vi "Puma_Ground_Control_Station.vi"(0 "?":refnum<visa-resource-name>="COM1", 1 "?":u32=9600, 9 "XON":u8=17 format="%.0x", 14 "XOFF":u8=19 format="%.0x", 15 "?":u32=10000, 21 "?":bool=TRUE, 24 "?":u8=10 format="%.0x", 25 "bsize":u32=4096) -> ()   [LabVIEW 2014]
doc: "The Advanced Serial Read and Write example performs a Serial Port Read, a Serial Port Write, or a combination of these actions while setting some advanced serial features like buffer size, termination characters, and XON/XOFF flow control. The user selects the actions (read or write) on the front panel. If both are selected, the VI will write the data first, read the data and then close the VISA session that is opened to the port. \n\nThe parameters set for the serial port must match the parameters of the connected instrument or device. In this example, the bytes to read parameter specifies the number of bytes that the serial port reads. If there were more bytes at the port than the number specified in bytes to read, those bytes would not be read. Also, if you specify to read more bytes than the number of bytes actually read, you might receive a timeout error message.\n\nINSTRUCTIONS:\n1) Select the serial resource and configuration parameters (baud rate, data bits, parity, stop bits, flow control).\n2) Termination character can be enabled and set. Also, set the required input buffer size prior to running the example.\n3) Select the operations to be performed. \n4) Connect the serial port to your device. If no device is available, perform a loopback test by doing one of the following. Short pins 2 and 3 on a RS-232 cable or short pin 4 to pin 8 and pin 5 to pin 9 on a RS-485/422 cable. \n5) Run the VI to see the data read. (The \"read string\" will match the \"string to write\" if a loopback test was performed.)\n\nThis example exposes several advanced features that you may need for your application. Not all applications need all the features shown in this example. The input buffer size is likely an important setting that you want to control in your application. This example expands upon the flow control option for XON and XOFF, allowing the user to choose those control characters. The timeout parameter has been brought to the front panel so a user can specify the time period the VISA Read will wait for the number of bytes to read before timing out. Also, the user has several controls for the termination character, which is discussed later.\n\nNote that you can press the write and read buttons and change the bytes to read parameters on the fly, while the example is running. However, you must stop the example to change the other configuration parameters after the example has started running, and then run again.\n\nSet the I/O buffer size slightly higher the amount of data you expect to receive. This is very important for applications that don't use flow control, as you may lose characters if the receive buffer overflows.\n\nSetting the timeout period ensures that the operation returns with a timeout error if the operation cannot be performed in the specified time period. \n\nSome devices require a termination character in order to identify the end of command strings. Some devices send a termination character to signify the end of data to be read. \n\nThis example shows how you can end the Read operation once a termination character is detected in the buffer and/or append a termination character at the end of the Write data. To enable the Read to end on a termination character, use the VISA Configure Serial Port or use the VISA Properties Serial End Mode for Reads, Termination Character Enable, and Termination Character. To end the Write with a termination character, use the VISA Properties Serial End Mode for Writes, the Send End Enable, and Termination Character. In this example, the same termination character is used for both the Read and the Write. You can specify two different characters for your application, if desired.\n\nYour application may require specific characters for the XON/XOFF Flow Control. You can specify these characters with the VISA Properties Flow Control XOFF Character and Flow Control XON Character. Note that if the standard XON and XOFF characters are used, then decimal 17 and 19 are unavailable for data values. Remember that using flow control and setting an adequate buffer size allow you to prevent buffer overflows."
uses:
  <vilib>/Instr/_visa.llb/VISA Configure Serial Port (Instr).vi
panel:
  out "soft kill ind":bool
  out "dump fuel ind":bool
  out "abort ind":bool
  out "run ind":bool
  out "av6-t ind":bool
  out "Control input":bool
  out "return yes on a completed input":bool
  out "Control (on/off)":bool
  out "PT 7":dbl
  out "PT7":dbl
  out "PT6":dbl
  out "PT5":dbl
  out "PT4":dbl
  out "PT3":dbl
  out "PT2":dbl
  out "PT1":dbl
  out "TC6":dbl
  out "TC5":dbl
  out "TC4":dbl
  out "TC3":dbl
  out "TC2":dbl
  out "TC1":dbl
  out "Output":string
  in  "?":enum32{"Check Out's", "Test"}(tab)
  in  "Tank ISO / AV5-T":bool
  in  "DValve / AV6-T":bool
  in  "Ullage ISO / FC-U":bool
  in  "UDump / FO-U":bool
  in  "Flight Control Board":bool
  in  "Safety":bool
  in  "Test Run":bool
  in  "Reset Control":bool
  in  "Primary Safety":bool
  out "?":bool
  out "?":bool
  out "?":bool
  out "?":bool
  in  "Primary Safety TEST Primary Safety":bool
  in  "Soft Kill":bool
  in  "Extra Switch":bool
  in  "Reset FC":bool
  in  "PixHawk":bool
  in  "Flight Control":bool
  in  "Safety":bool
  in  "Takeoff":bool
  in  "abort":bool
  out "?":dbl(graph)
  in  "Send Command":bool=TRUE
  in  "Manual":string="*IDN?"
  in  "?":bool=TRUE
  in  "bytes to read 2":u32=1000
  out "?":u32
  out "?":string[](array[string])
  out "?":string[](array[string])
  out "?":T1(graph)
  out "Voltage Sensor":dbl
  out "PT 1":dbl
  out "PT 2":dbl
  out "PT 3":dbl
  out "PT 4":dbl
  out "PT 5":dbl
  out "PT 6":dbl
  out "TC 1":dbl
  out "TC 2":dbl
  out "TC 3":dbl
  out "TC 4":dbl
  out "TC 5":dbl
  out "TC 6":dbl
  in  "dump fuel":bool
  in  "?":enum32{"PT", "TC", "Test"}(tab)
  in  "?":T2(tab)
  out "PT 1":dbl(graph)
  out "PT 2":dbl(graph)
  out "PT 3":dbl(graph)
  out "PT 4":dbl(graph)
  out "PT 5":dbl(graph)
  out "PT 6":dbl(graph)
  out "PT 7":dbl(graph)
  in  "?":T3(tab)
  out "TC 1":dbl(graph)
  out "TC 2":dbl(graph)
  out "TC 3":dbl(graph)
  out "TC 4":dbl(graph)
  out "TC 5":dbl(graph)
  out "TC 6":dbl(graph)
  out "?":bool
  out "String":string
  in  "String 3":string
  in  "Turn Off":bool
  in  "?":bool=TRUE
  in  "?":bool
  in  "Av-6Tt":bool
  in  "?":bool
  in  "?":bool
  out "AV4-T":bool
  out "AV3-T":bool
  out "AV2-T":bool
  out "AV1-T":bool
  out "AV6-T":bool
  out "AV5-T":bool
  out "FO-U":bool
  out "FC-U":bool
  out "?":dbl(slide) scale=0.2..200.0
  # "FC-U"
  # "FO-U"
  # "AV1-T"
  # "AV2-T"
  # "AV3-T"
  # "AV4-T"
  # "AV5-T"
  # "AV6-T"
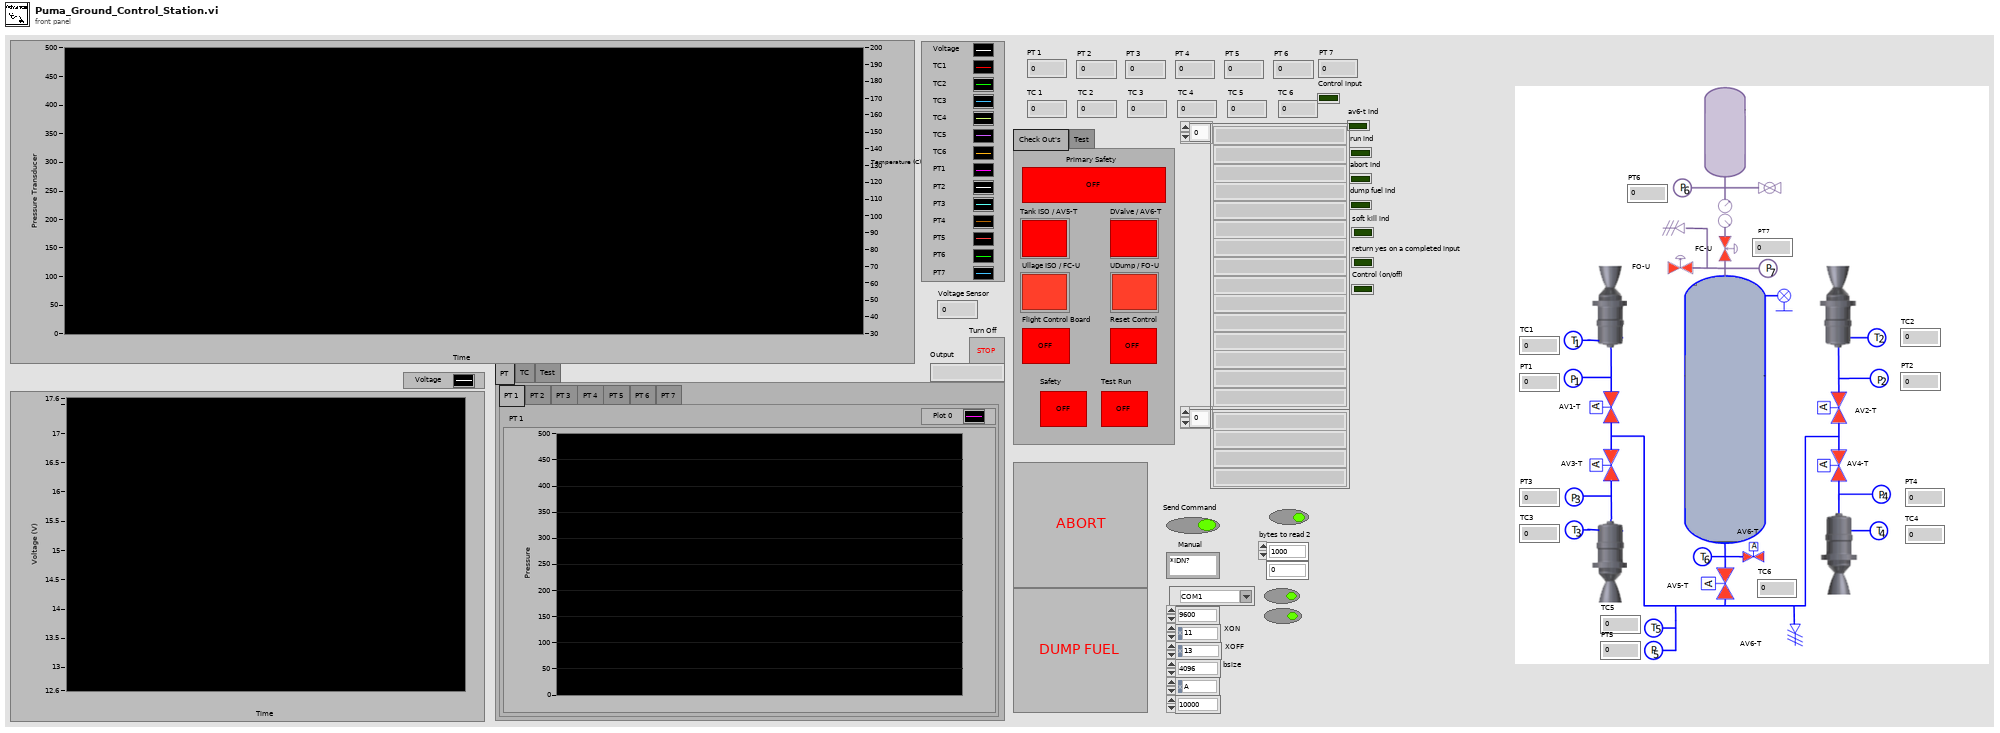
[diagram p1: front panel]
types:
  T1 = cluster{dbl, dbl, dbl, dbl, dbl, dbl, dbl, dbl, dbl, dbl, dbl, dbl, dbl, dbl}
  T2 = enum32{"PT 1", "PT 2", "PT 3", "PT 4", "PT 5", "PT 6", "PT 7"}
  T3 = enum32{"TC 1", "TC 2", "TC 3", "TC 4", "TC 5", "TC 6"}
  T4 = cluster{"Read Access":enum8{"Allowed", "Required", "None"}, "Write Access":enum8{"Allowed", "Required", "None"}}
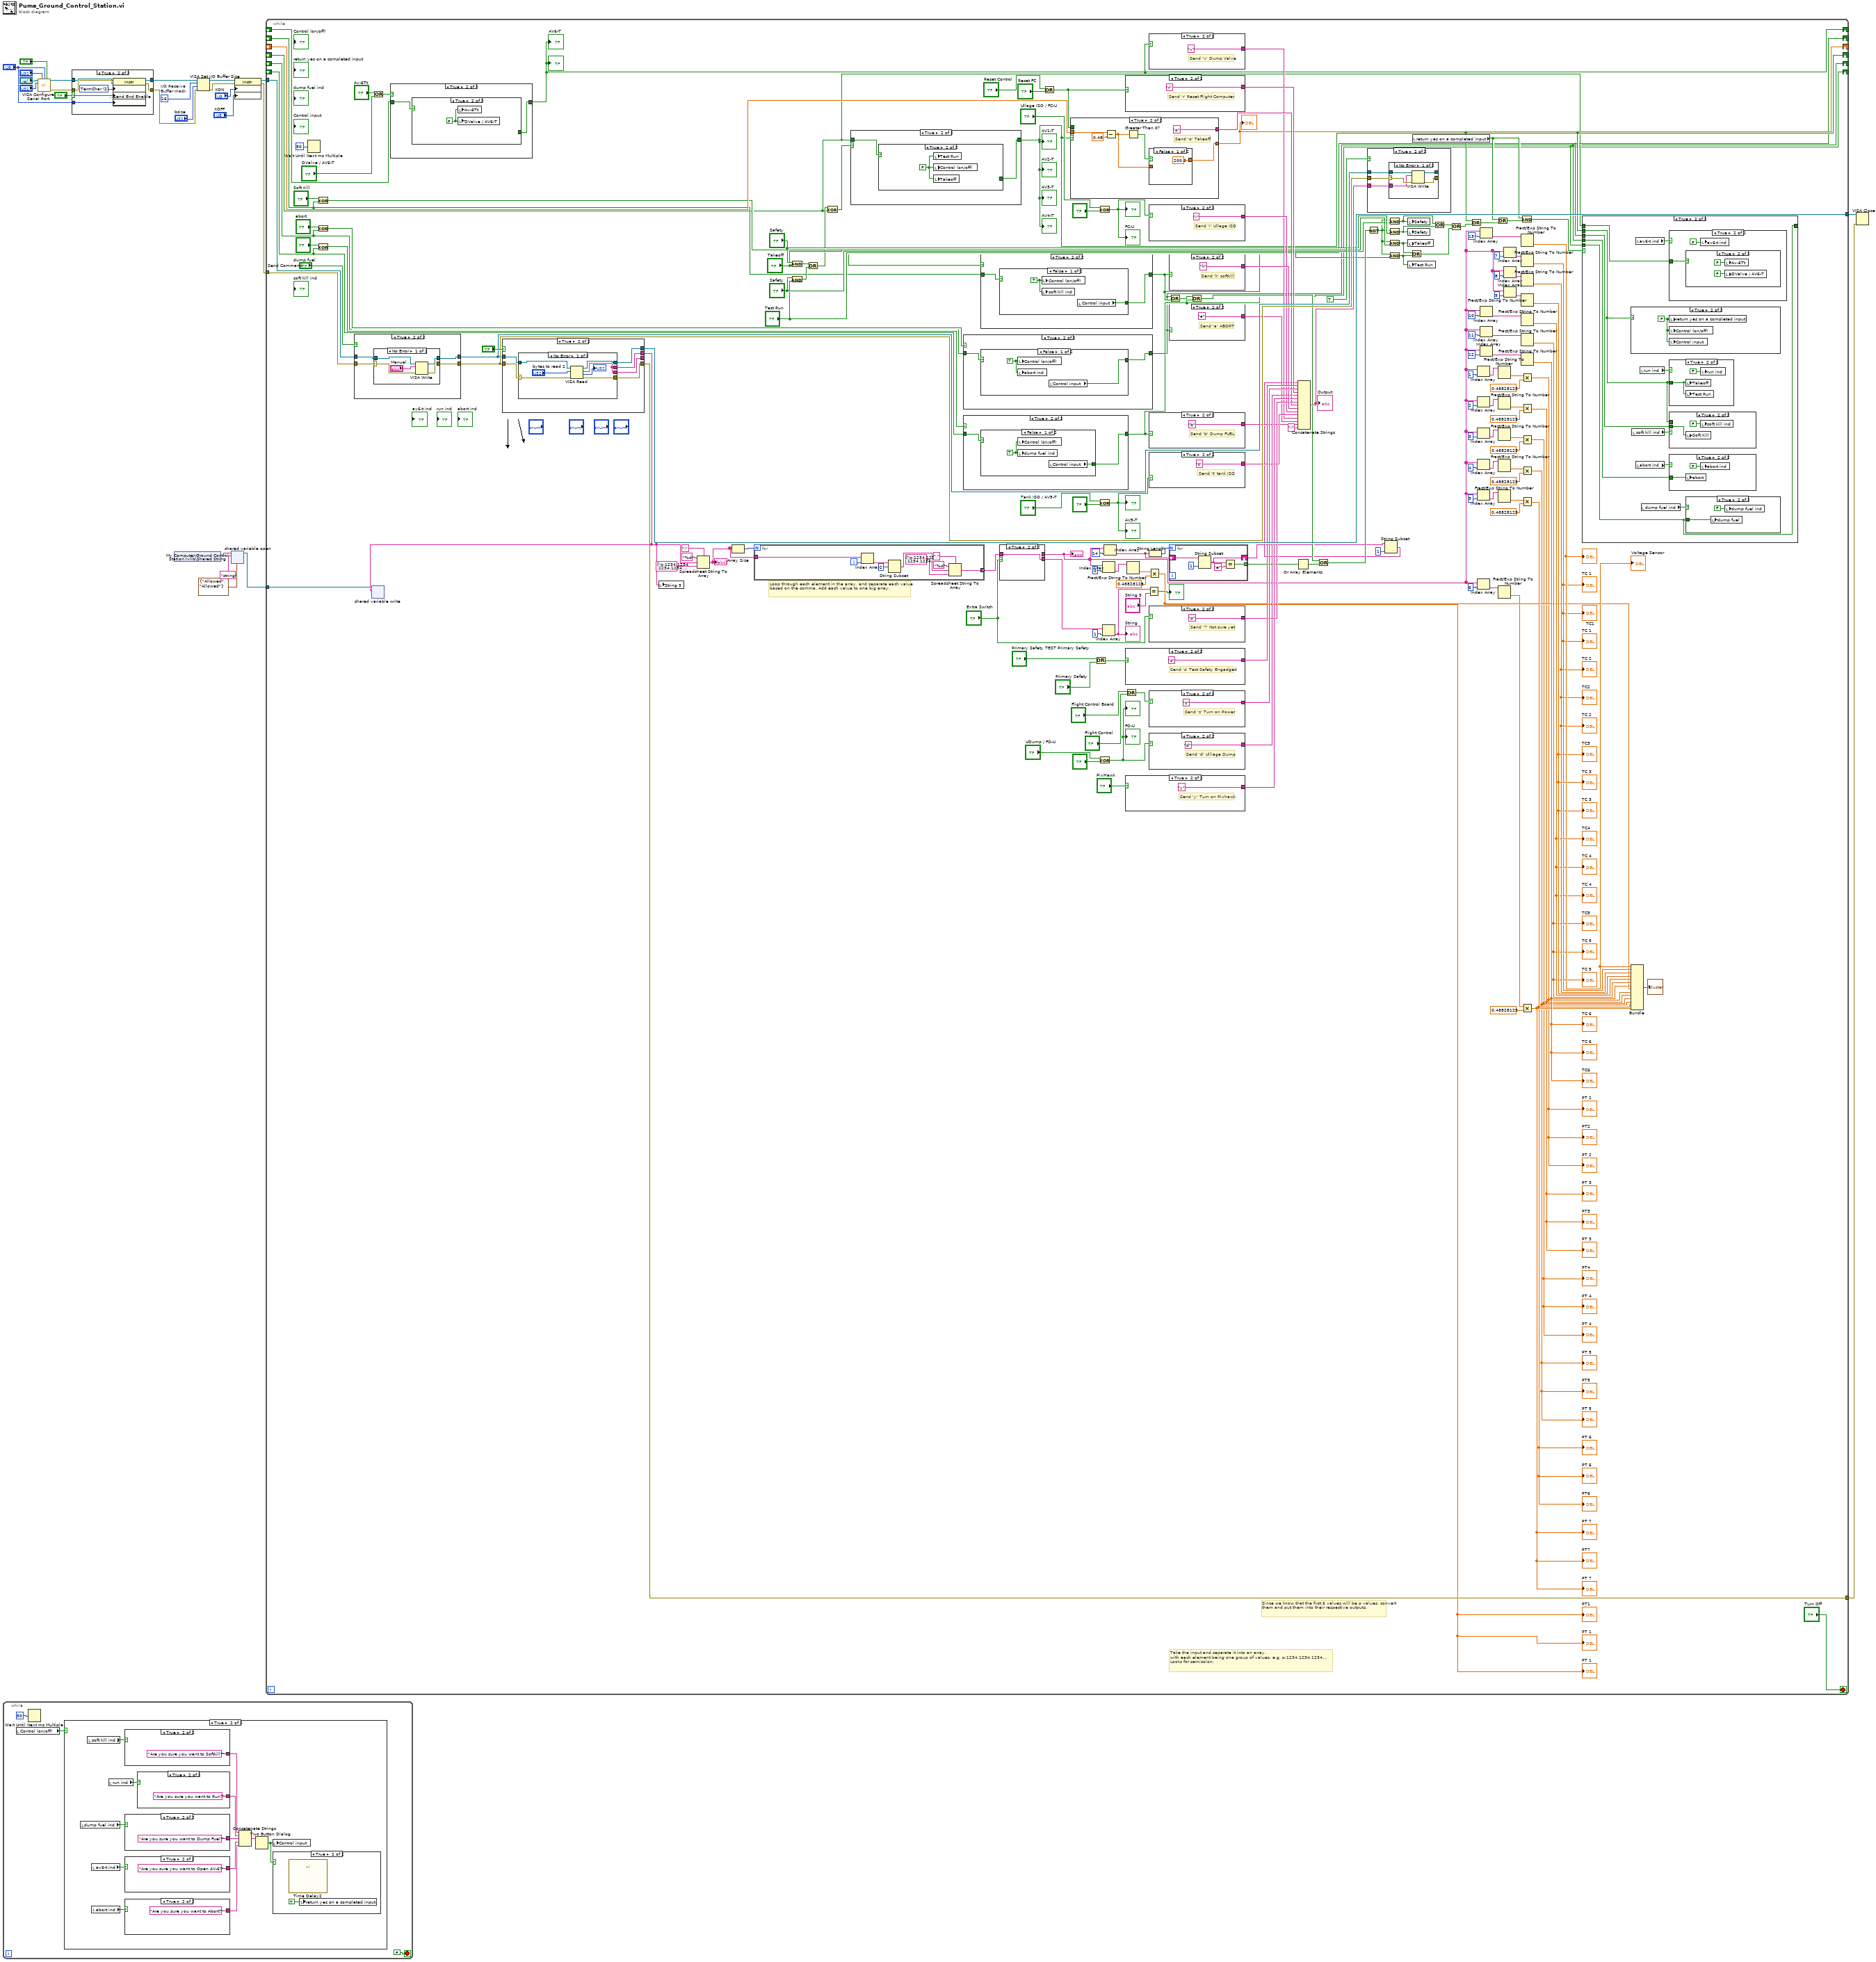
[diagram p0: block diagram]
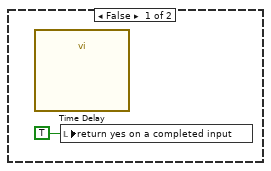
[diagram p8: hidden frame]
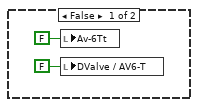
[diagram p11: hidden frame]
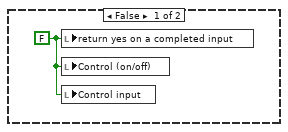
[diagram p16: hidden frame]
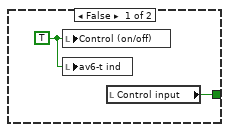
[diagram p18: hidden frame]
diagram:
  w20 = u16 16  # I/O Receive Buffer mask
  n1 = while {
    stop <- FALSE stop-if-true
    n2 = local read "Control (on/off)"() -> (w27:bool)
    n3 = Wait Until Next ms Multiple(millisecond multiple=u32 50 ("milliseconds to wait")) -> ()  [unwired: 1 out]
    n4 = case shown="True" w27 {
      frame False {
      }
      frame True {
        n5 = local read "dump fuel ind"() -> (w36:bool)
        n6 = local read "soft kill ind"() -> (w34:bool)
        n7 = local read "av6-t ind"() -> (w37:bool)
        n8 = local read "abort ind"() -> (w38:bool)
        n9 = local read "run ind"() -> (w35:bool)
        n10 = case shown="True" w34 {
          tunnel: [_ "Are you sure you want to Softkill?"] -> w29
          frame False {
          }
          frame True {
          }
        }
        n11 = case shown="True" w36 {
          tunnel: [_ "Are you sure you want to Dump Fuel?"] -> w31
          frame False {
          }
          frame True {
          }
        }
        n12 = case shown="True" w37 {
          tunnel: [_ "Are you sure you want to Open AV-6?"] -> w32
          frame False {
          }
          frame True {
          }
        }
        n13 = case shown="True" w38 {
          tunnel: [_ "Are you sure you want to Abort?"] -> w33
          frame False {
          }
          frame True {
          }
        }
        n14 = case shown="True" w35 {
          tunnel: [_ "Are you sure you want to Run?"] -> w30
          frame False {
          }
          frame True {
          }
        }
        n15 = Concatenate Strings(w29, w30, w31, w32, w33) -> (w28:string)
        n16 = Two Button Dialog(message=w28) -> (T button?=w39:bool)  [unwired: 2 in]
        n17 = local write "Control input"(w39) -> ()
        n18 = case shown="True" w39 {
          frame False {
            n19 = call "Time Delay"() -> ()  [unwired: 11 in, 1 out]
            n20 = local write "return yes on a completed input"(TRUE) -> ()
          }
          frame True {
            n21 = call "Time Delay2"() -> ()  [unwired: 11 in, 1 out]
            n22 = local write "return yes on a completed input"(TRUE) -> ()
          }
        }
      }
    }
  }
  n23 = call-poly "VISA Configure Serial Port"("VISA resource name"="?", "timeout (10sec)"="?", "termination char\n(0xA = '\\n' = LF)"="?", "Enable Termination\nChar (T)"="?", "baud rate (9600)"="?") -> ("VISA resource name out"=w9:refnum<visa-resource-name>, "error out"=w12:errorcluster)  [unwired: 5 in, 4 out]
  n24 = case shown="True" "?" {
    selector: "?" -> [_ w49]
    tunnel: w9 -> [w47 w55]
    tunnel: w12 -> [w48 w54]
    tunnel: [w47 w53] -> w10
    tunnel: [w48 w52] -> w11
    tunnel: "?" -> [_ w50]
    frame False {
    }
    frame True {
      w51 = u16 2 items=["None", "LastBit", "TermChar", "Break"] ("Serial Settings:Serial End Mode for Writes")
      n25 = property class="Instr"(reference=w55, error in=w54, "Serial Settings:End Mode for Writes"=w51, "Message Based Settings:Send End Enable"=w49, "Message Based Settings:Termination Character"=w50) -> (reference out=w53:refnum<visa-resource-name>, error out=w52:errorcluster)
    }
  }
  n26 = shared-variable "My Computer\\Ground Control Station.lvlib\\Shared String"() -> (w2:string)  [unwired: 1 in, 1 out]
  n27 = VISA Set I/O Buffer Size(VISA resource name=w10, mask (16)=w20, size (4096)="bsize", error in (no error)=w11) -> (VISA resource name out=w16:refnum<visa-resource-name>, error out=w15:errorcluster)
  n28 = shared-variable-open(w2, "string", T4 {"Read Access"=enum."Allowed", "Write Access"=enum."Allowed"} ("access")) -> (w1:refnum<k21>)  [unwired: 1 in, 1 out]
  n29 = property class="Instr"(reference=w16, error in=w15, "Serial Settings:Flow Control XON Character"="XON", "Serial Settings:Flow Control XOFF Character"="XOFF") -> (reference out=w8:refnum<visa-resource-name>, error out=w7:errorcluster)
  n30 = while {
    tunnel: w8 -> [w191]
    tunnel: w7 -> [w190]
    tunnel: [w189] -> w6
    tunnel: [w58] -> w5
    shift-right: [w149] -> _
    shift-left: _ -> [w148]
    shift-right: [w84] -> _
    shift-left: _ -> [w66]
    shift-right: [w74] -> _
    shift-left: _ -> [w75]
    shift-right: [w64] -> _
    shift-left: _ -> [w91]
    shift-right: [w65] -> _
    shift-left: _ -> [w88]
    shift-right: [w67] -> _
    shift-left: _ -> [w70]
    tunnel: w1 -> [w57]
    stop <- "Turn Off" stop-if-true
    # "Since we know that the first 6 values will be p values, convert them and put them into their respective outputs."
    # "Loop through each element in the array, and separate each value\nbased on the comma. Add each value to one big array."
    # "Take the input and separate it into an array,\nwith each element being one group of values, e.g. p:1234,1234,1234...\nLooks for semicolon."
    n31 = Wait Until Next ms Multiple(millisecond multiple=u32 50 ("milliseconds to wait")) -> ()  [unwired: 1 out]
    n32 = Exclusive Or(1:w70, 2:"Soft Kill") -> (0:w68:bool)
    n33 = Exclusive Or(1:w91, 2:"abort") -> (0:w93:bool)
    n34 = Exclusive Or(1:w88, 2:"dump fuel") -> (0:w90:bool)
    n35 = case shown="True" "Send Command" {
      tunnel: [w322 w326] -> w184
      tunnel: [w321 w325] -> w183
      tunnel: w191 -> [w322 w324]
      tunnel: w190 -> [w321 w323]
      frame False {
      }
      frame True {
        n36 = case shown="No Error" w323 {
          selector: w323 -> [w327 w333]
          tunnel: [w331 w332] -> w326
          tunnel: [w330 w333] -> w325
          tunnel: w324 -> [w328 w332]
          frame No Error {
            n37 = VISA Write(VISA resource name=w328, write buffer="Manual", error in (no error)=w327) -> (VISA resource name out=w331:refnum<visa-resource-name>, error out=w330:errorcluster)  [unwired: 1 out]
          }
          frame Error {
          }
        }
      }
    }
    n38 = Or(x="Av-6Tt", y="DValve / AV6-T") -> (x .or. y?=w71:bool)
    n39 = case shown="True" w71 {
      tunnel: [w251 w252] -> w74
      tunnel: w75 -> [w251 w253]
      frame False {
      }
      frame True {
        n40 = case shown="True" w253 {
          tunnel: [w255 _] -> w252
          frame False {
            w254 = TRUE
            n41 = local write "Control (on/off)"(w254) -> ()
            n42 = local write "av6-t ind"(w254) -> ()
            n43 = local read "Control input"() -> (w255:bool)
          }
          frame True {
            w256 = FALSE
            n44 = local write "Av-6Tt"(w256) -> ()
            n45 = local write "DValve / AV6-T"(w256) -> ()
          }
        }
      }
    }
    "AV6-T" <- w74
    "?" <- w74
    n46 = case shown="True" "?" {
      tunnel: w183 -> [w334 w339]
      tunnel: w184 -> [w335 w338]
      tunnel: [w334 w341] -> w58
      tunnel: [w335 w340] -> w189
      tunnel: [_ w337] -> _
      tunnel: [_ w336] -> w56
      frame False {
      }
      frame True {
        n47 = case "Read bytes from port." shown="No Error" w339 {
          selector: w339 -> [w344 w349]
          tunnel: [w347 w349] -> w341
          tunnel: [w348 w350] -> w340
          tunnel: w338 -> [w345 w350]
          tunnel: [w342 _] -> w337
          tunnel: [w342 _] -> w336
          frame No Error {
            n48 = VISA Read(VISA resource name=w345, byte count="bytes to read 2", error in (no error)=w344) -> (VISA resource name out=w348:refnum<visa-resource-name>, read buffer=w342:string, return count=→"?":u32, error out=w347:errorcluster)
          }
          frame Error {
            # "Error occurred \nreading Bytes at \nSerial Port"
          }
        }
      }
    }
    n49 = shared-variable-write(w57, w56) -> ()  [unwired: 1 in, 2 out]
    n50 = local write "String 3"(w56) -> ()
    n51 = Spreadsheet String To Array(delimiter (Tab)=";", format string="%d", spreadsheet string=w56, array type (2D Dbl)=string[] ["p:1234.1234.1234.1234,1234,1234", "t:1234,1234,1234"] ("Array of Strings 3")) -> (array=w217:string[])
    "?" <- w217
    n52 = Array Size(array=w217) -> (size(s)=w218:i32)
    n53 = for {
      N: w218 -> [_]
      tunnel: w217 -> [w359]
      tunnel: [w351] -> w112 mode=concatenating
      i -> [w358]
      n54 = Index Array(array=w359, index=w358) -> (element=w354:string)
      n55 = String Subset(string=w354, offset (0)=2) -> (substring=w352:string)  [unwired: 1 in]
      n56 = Spreadsheet String To Array(delimiter (Tab)=",", format string="%d", spreadsheet string=w352, array type (2D Dbl)=string[] ["p:1234.1234.1234.1234,1234,1234", "t:1234,1234,1234"] ("Array of Strings 3")) -> (array=w351:string[])
    }
    n57 = And(x="Safety", y="Takeoff") -> (x .and. y?=w169:bool)
    n58 = And(x="Safety", y="Test Run") -> (x .and. y?=w170:bool)
    n59 = Or(x=w169, y=w170) -> (x .or. y?=w96:bool)
    n60 = Exclusive Or(1:w66, 2:w96) -> (0:w95:bool)
    n61 = case shown="True" w95 {
      tunnel: [w273 w275] -> w84
      tunnel: w66 -> [w273 w274]
      frame False {
      }
      frame True {
        n62 = case shown="True" w274 {
          tunnel: [w277 _] -> w275
          frame False {
            w276 = TRUE
            n63 = local write "Control (on/off)"(w276) -> ()
            n64 = local write "run ind"(w276) -> ()
            n65 = local read "Control input"() -> (w277:bool)
          }
          frame True {
            w278 = FALSE
            n66 = local write "Test Run"(w278) -> ()
            n67 = local write "Control (on/off)"(w278) -> ()
            n68 = local write "Takeoff"(w278) -> ()
          }
        }
      }
    }
    "AV1-T" <- w84
    "AV4-T" <- w84
    "AV2-T" <- w84
    "AV3-T" <- w84
    n69 = case shown="True" w93 {
      tunnel: [w267 w269] -> w64
      tunnel: w91 -> [w267 w268]
      frame False {
      }
      frame True {
        n70 = case shown="False" w268 {
          tunnel: [w270 FALSE ("T button?")] -> w269
          frame False {
            w271 = TRUE
            n71 = local write "Control (on/off)"(w271) -> ()
            n72 = local write "abort ind"(w271) -> ()
            n73 = local read "Control input"() -> (w270:bool)
          }
          frame True {
          }
        }
      }
    }
    n74 = case shown="True" w90 {
      tunnel: [w262 w264] -> w65
      tunnel: w88 -> [w262 w263]
      frame False {
      }
      frame True {
        n75 = case shown="False" w263 {
          tunnel: [w266 _] -> w264
          frame False {
            w265 = TRUE
            n76 = local write "Control (on/off)"(w265) -> ()
            n77 = local write "dump fuel ind"(w265) -> ()
            n78 = local read "Control input"() -> (w266:bool)
          }
          frame True {
          }
        }
      }
    }
    n79 = case shown="True" w68 {
      tunnel: [w257 w259] -> w67
      tunnel: w70 -> [w257 w258]
      frame False {
      }
      frame True {
        n80 = case shown="False" w258 {
          tunnel: [w260 _] -> w259
          frame False {
            w261 = TRUE
            n81 = local write "Control (on/off)"(w261) -> ()
            n82 = local write "soft kill ind"(w261) -> ()
            n83 = local read "Control input"() -> (w260:bool)
          }
          frame True {
          }
        }
      }
    }
    n84 = case shown="True" "Extra Switch" {
      tunnel: w112 -> [w284 w285]
      tunnel: [w284 _] -> w114
      tunnel: [_ w285] -> w111
      frame False {
      }
      frame True {
      }
    }
    "?" <- w114
    n85 = Or(x="Reset Control", y="Reset FC") -> (x .or. y?=w150:bool)
    n86 = case shown="True" w84 {
      tunnel: [_ "o" ("write buffer")] -> w175
      tunnel: w148 -> [w295 w303]
      tunnel: [w296 w299] -> w149
      tunnel: w150 -> [w294 _]
      frame False {
        n87 = case shown="False" w294 {
          tunnel: [w297 200.0] -> w296
          tunnel: w295 -> [w297 _]
          frame False {
          }
          frame True {
          }
        }
      }
      frame True {
        # "Send 'o' Takeoff"
        n88 = Subtract(x=w303, y=0.48) -> (x-y=w300:dbl)
        n89 = Greater Than 0?(x=w300) -> (x > 0?=w301:bool)
        n90 = case shown="False" w301 {
          tunnel: w300 -> [_ w306]
          tunnel: [200.0 w306] -> w299
          frame False {
          }
          frame True {
          }
        }
      }
    }
    "?" <- w149
    n91 = Or(x="Primary Safety TEST Primary Safety", y="Primary Safety") -> (x .or. y?=w136:bool)
    n92 = Exclusive Or(1:"?", 2:"Ullage ISO / FC-U") -> (0:w139:bool)
    "FC-U" <- w139
    "?" <- w139
    n93 = Exclusive Or(1:"?", 2:"Tank ISO / AV5-T") -> (0:w142:bool)
    "AV5-T" <- w142
    "?" <- w142
    n94 = Exclusive Or(1:"?", 2:"UDump / FO-U") -> (0:w145:bool)
    "FO-U" <- w145
    "?" <- w145
    n95 = Index Array(array=w114, index=0) -> (element=w210:string)
    n96 = Index Array(array=w111, index=1) -> (element=w110:string)
    "String" <- w110
    n97 = Index Array(array=w114, index=14) -> (element=w59:string)
    n98 = case shown="True" w150 {
      tunnel: [_ "r" ("write buffer")] -> w179
      frame False {
      }
      frame True {
        # "Send 'r' Reset Flight Computer"
      }
    }
    n99 = case shown="True" w136 {
      tunnel: [_ "s" ("write buffer")] -> w182
      frame False {
      }
      frame True {
        # "Send 's' Test Safety Engadged"
      }
    }
    n100 = case shown="True" "PixHawk" {
      tunnel: [_ "y" ("write buffer")] -> w177
      frame False {
      }
      frame True {
        # "Send 'y' Turn on Pixhawk"
      }
    }
    n101 = Or(x="Flight Control Board", y="Flight Control") -> (x .or. y?=w166:bool)
    n102 = Fract/Exp String To Number(string=w210) -> (number=w131:dbl)  [unwired: 3 in, 1 out]
    n103 = Equal?(x=w110, y="String 3") -> (x = y?=→"?":bool)
    n104 = Multiply(x=w131, y=0.48828125) -> (x*y=w130:dbl)
    "PT 1" <- w130
    "PT 1" <- w130
    "PT1" <- w130
    n105 = case shown="True" w74 {
      tunnel: [_ "v" ("write buffer")] -> w162
      frame False {
      }
      frame True {
        # "Send 'v' Dump Valve"
      }
    }
    n106 = case shown="True" w139 {
      tunnel: [_ "i" ("write buffer")] -> w164
      frame False {
      }
      frame True {
        # "Send 'i' Ullage ISO"
      }
    }
    n107 = case shown="True" w65 {
      tunnel: [_ "b" ("write buffer")] -> w161
      frame False {
      }
      frame True {
        # "Send 'b' Dump FUEL"
      }
    }
    n108 = case shown="True" w142 {
      tunnel: [_ "t" ("write buffer")] -> w163
      frame False {
      }
      frame True {
        # "Send 't' tank ISO"
      }
    }
    n109 = String Length(string=w59) -> (length=w106:i32)
    n110 = case shown="True" "Extra Switch" {
      tunnel: [_ "p" ("write buffer")] -> w176
      frame False {
      }
      frame True {
        # "Send '?' Not sure yet"
      }
    }
    n111 = case shown="True" w166 {
      tunnel: [_ "z" ("write buffer")] -> w180
      frame False {
      }
      frame True {
        # "Send 'z' Turn on Power"
      }
    }
    n112 = case shown="True" w145 {
      tunnel: [_ "d" ("write buffer")] -> w165
      frame False {
      }
      frame True {
        # "Send 'd' Ulliage Dump"
      }
    }
    n113 = case shown="True" w67 {
      tunnel: [_ "k" ("write buffer")] -> w178
      frame False {
      }
      frame True {
        # "Send 'k' softkill"
      }
    }
    n114 = Or(x=w64, y=w67) -> (x .or. y?=w94:bool)
    n115 = case shown="True" w64 {
      tunnel: [_ "a" ("write buffer")] -> w160
      frame False {
      }
      frame True {
        # "Send 'a' ABORT"
      }
    }
    n116 = for {
      N: w106 -> [_]
      shift-right: [w281] -> w61
      shift-left: w59 -> [w280]
      tunnel: [w279] -> w105 mode=indexing
      n117 = String Subset(string=w280, length (rest)=1 ("length (rest)")) -> (substring=w281:string)  [unwired: 1 in]
      n118 = Equal?(x=w281, y="e") -> (x = y?=w279:bool)
    }
    n119 = Or(x=w94, y=w65) -> (x .or. y?=w103:bool)
    n120 = Or Array Elements(Boolean array=w105) -> (logical OR=w104:bool)
    n121 = Or(x=w103, y=w104) -> (x .or. y?=w102:bool)
    n122 = Not(x=w102) -> (.not. x?=w98:bool)
    n123 = String Subset(string=w61, length (rest)=1 ("length (rest)")) -> (substring=w63:string)  [unwired: 1 in]
    n124 = Concatenate Strings(w63, w182, w180, w179, w165, w177, w176, w175, w178, w164, w163, w162, w160, w161, ";" ("string")) -> (w173:string)
    "Output" <- w173
    n125 = case shown="True" TRUE {
      tunnel: w184 -> [_ w313]
      tunnel: w183 -> [_ w312]
      tunnel: w173 -> [_ w311]
      frame False {
      }
      frame True {
        n126 = case shown="No Error" w312 {
          selector: w312 -> [w315 w320]
          tunnel: [w318 w319] -> _
          tunnel: [w317 w320] -> _
          tunnel: w313 -> [w316 w319]
          tunnel: w311 -> [w314 _]
          frame No Error {
            n127 = VISA Write(VISA resource name=w316, write buffer=w314, error in (no error)=w315) -> (VISA resource name out=w318:refnum<visa-resource-name>, error out=w317:errorcluster)  [unwired: 1 out]
          }
          frame Error {
          }
        }
      }
    }
    n128 = And(x=w98, y="Safety") -> (x .and. y?=w79:bool)
    n129 = And(x=w98, y="Safety") -> (x .and. y?=w78:bool)
    n130 = And(x=w98, y="Takeoff") -> (x .and. y?=w77:bool)
    n131 = And(x=w98, y="Test Run") -> (x .and. y?=w76:bool)
    n132 = local write "Safety"(w79) -> ()
    n133 = local write "Safety"(w78) -> ()
    n134 = local write "Takeoff"(w77) -> ()
    n135 = local write "Test Run"(w76) -> ()
    n136 = Or(x=w77, y=w76) -> (x .or. y?=w81:bool)
    n137 = local read "return yes on a completed input"() -> (w86:bool)
    n138 = Or(x=w79, y=w78) -> (x .or. y?=w82:bool)
    n139 = Or(x=w82, y=w81) -> (x .or. y?=w80:bool)
    n140 = Or(x=w84, y=w80) -> (x .or. y?=w83:bool)
    n141 = Index Array(array=w114, index=1) -> (element=w209:string)
    n142 = Index Array(array=w114, index=2) -> (element=w208:string)
    n143 = Index Array(array=w114, index=3) -> (element=w207:string)
    n144 = Index Array(array=w114, index=4) -> (element=w206:string)
    n145 = Index Array(array=w114, index=5) -> (element=w205:string)
    n146 = Index Array(array=w114, index=6) -> (element=w152:string)
    n147 = Index Array(array=w114, index=13) -> (element=w187:string)
    n148 = Index Array(array=w114, index=10) -> (element=w195:string)
    n149 = Index Array(array=w114, index=11) -> (element=w194:string)
    n150 = Index Array(array=w114, index=12) -> (element=w193:string)
    n151 = Or(x=w86, y=w83) -> (x .or. y?=w87:bool)
    n152 = Fract/Exp String To Number(string=w209) -> (number=w116:dbl)  [unwired: 3 in, 1 out]
    n153 = Fract/Exp String To Number(string=w208) -> (number=w119:dbl)  [unwired: 3 in, 1 out]
    n154 = Fract/Exp String To Number(string=w207) -> (number=w122:dbl)  [unwired: 3 in, 1 out]
    n155 = Fract/Exp String To Number(string=w206) -> (number=w125:dbl)  [unwired: 3 in, 1 out]
    n156 = Fract/Exp String To Number(string=w205) -> (number=w134:dbl)  [unwired: 3 in, 1 out]
    n157 = Fract/Exp String To Number(string=w152) -> (number=w128:dbl)  [unwired: 3 in, 1 out]
    n158 = Index Array(array=w114, index=7) -> (element=w199:string)
    n159 = Index Array(array=w114, index=8) -> (element=w198:string)
    n160 = Index Array(array=w114, index=9) -> (element=w197:string)
    n161 = And(x=w86, y=w87) -> (x .and. y?=w85:bool)
    n162 = Fract/Exp String To Number(string=w187) -> (number=w186:dbl)  [unwired: 3 in, 1 out]
    "Voltage Sensor" <- w186
    "?" <- w186
    n163 = Fract/Exp String To Number(string=w199) -> (number=w153:dbl)  [unwired: 3 in, 1 out]
    "TC 1" <- w153
    "TC 1" <- w153
    "TC1" <- w153
    n164 = Fract/Exp String To Number(string=w198) -> (number=w158:dbl)  [unwired: 3 in, 1 out]
    "TC 2" <- w158
    "TC 2" <- w158
    "TC2" <- w158
    n165 = Fract/Exp String To Number(string=w197) -> (number=w157:dbl)  [unwired: 3 in, 1 out]
    "TC 3" <- w157
    "TC 3" <- w157
    "TC3" <- w157
    n166 = Fract/Exp String To Number(string=w195) -> (number=w156:dbl)  [unwired: 3 in, 1 out]
    "TC 4" <- w156
    "TC 4" <- w156
    "TC4" <- w156
    n167 = Fract/Exp String To Number(string=w194) -> (number=w155:dbl)  [unwired: 3 in, 1 out]
    "TC 5" <- w155
    "TC 5" <- w155
    "TC5" <- w155
    n168 = Fract/Exp String To Number(string=w193) -> (number=w154:dbl)  [unwired: 3 in, 1 out]
    "TC 6" <- w154
    "TC 6" <- w154
    "TC6" <- w154
    n169 = Multiply(x=w116, y=0.48828125) -> (x*y=w115:dbl)
    "PT 2" <- w115
    "PT 2" <- w115
    "PT2" <- w115
    n170 = Multiply(x=w119, y=0.48828125) -> (x*y=w118:dbl)
    "PT 3" <- w118
    "PT 3" <- w118
    "PT3" <- w118
    n171 = Multiply(x=w122, y=0.48828125) -> (x*y=w121:dbl)
    "PT 4" <- w121
    "PT 4" <- w121
    "PT4" <- w121
    n172 = Multiply(x=w125, y=0.48828125) -> (x*y=w124:dbl)
    "PT 5" <- w124
    "PT 5" <- w124
    "PT5" <- w124
    n173 = Multiply(x=w134, y=0.48828125) -> (x*y=w133:dbl)
    "PT 6" <- w133
    "PT 6" <- w133
    "PT6" <- w133
    n174 = Multiply(x=w128, y=0.48828125) -> (x*y=w127:dbl)
    "PT7" <- w127
    "PT 7" <- w127
    "PT 7" <- w127
    n175 = case shown="True" w85 {
      tunnel: w84 -> [_ w226]
      tunnel: w67 -> [_ w229]
      tunnel: w66 -> [_ w228]
      tunnel: [_ w227] -> _
      tunnel: w65 -> [_ w227]
      tunnel: w64 -> [_ w225]
      frame False {
      }
      frame True {
        n176 = case shown="True" w226 {
          frame False {
            w249 = FALSE
            n177 = local write "return yes on a completed input"(w249) -> ()
            n178 = local write "Control (on/off)"(w249) -> ()
            n179 = local write "Control input"(w249) -> ()
          }
          frame True {
            w250 = FALSE
            n180 = local write "return yes on a completed input"(w250) -> ()
            n181 = local write "Control (on/off)"(w250) -> ()
            n182 = local write "Control input"(w250) -> ()
          }
        }
        n183 = local read "soft kill ind"() -> (w234:bool)
        n184 = local read "av6-t ind"() -> (w230:bool)
        n185 = local read "abort ind"() -> (w231:bool)
        n186 = local read "run ind"() -> (w232:bool)
        n187 = local read "dump fuel ind"() -> (w233:bool)
        n188 = case shown="True" w230 {
          tunnel: w228 -> [_ w236]
          frame False {
          }
          frame True {
            n189 = case shown="True" w236 {
              frame False {
                n190 = local write "Av-6Tt"(FALSE) -> ()
                n191 = local write "DValve / AV6-T"(FALSE) -> ()
              }
              frame True {
                n192 = local write "Av-6Tt"(FALSE) -> ()
                n193 = local write "DValve / AV6-T"(FALSE) -> ()
              }
            }
            n194 = local write "av6-t ind"(FALSE) -> ()
          }
        }
        n195 = case shown="True" w232 {
          tunnel: w226 -> [_ w248]
          frame False {
          }
          frame True {
            n196 = local write "Takeoff"(w248) -> ()
            n197 = local write "Test Run"(w248) -> ()
            n198 = local write "run ind"(FALSE) -> ()
          }
        }
        n199 = case shown="True" w234 {
          tunnel: w226 -> [_ _]
          tunnel: w229 -> [_ w243]
          frame False {
          }
          frame True {
            n200 = local write "Soft Kill"(w243) -> ()
            n201 = local write "soft kill ind"(FALSE) -> ()
          }
        }
        n202 = case shown="True" w231 {
          tunnel: w225 -> [_ w241]
          frame False {
          }
          frame True {
            n203 = local write "abort"(w241) -> ()
            n204 = local write "abort ind"(FALSE) -> ()
          }
        }
        n205 = case shown="True" w233 {
          tunnel: w227 -> [_ w245]
          frame False {
          }
          frame True {
            n206 = local write "dump fuel"(w245) -> ()
            n207 = local write "dump fuel ind"(FALSE) -> ()
          }
        }
      }
    }
    n208 = Bundle(w186, w153, w158, w157, w156, w155, w154, w130, w115, w118, w121, w124, w133, w127) -> (→"?":T1)  [unwired: 1 out]
  }
  n209 = VISA Close(VISA resource name=w6, error in (no error)=w5) -> ()  [unwired: 1 out]
